vi "Launch DQMH Tools by menu.vi"(8 "error in":errorcluster, 11 "DQMH Tools":T1) -> (0 "error out":errorcluster)   [LabVIEW 2020]
doc: "Launch a DQMH scripting tool by typing one of the following strings in Quick Drop before pressing the Ctrl-Key shortcut for this plugin:\n\nCreate New DQMH Event - ae, new event, add event, create event, \"\" (empty string)\nRename DQMH Event - re, rename event\nRemove DQMH Event - rme, remove\nConvert DQMH Event - ce, convert\nAdd New DQMH Module - am, new mod, add mod, create mod\nRename DQMH Module - rm, rename module\nValidate DQMH Module - vm, validate\nCreate DQMH Module Template - ct, template\nCreate RT Tester - crt, rt\nNew DQMH Unit Test - cut, unit\n\nDefault Shortcut - [E]"
uses:
  controls/DQMH Tools Menu--enum.ctl
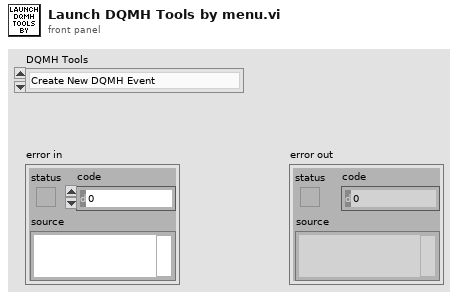
[diagram p1: front panel]
types:
  T1 = typedef "DQMH Tools Menu--enum.ctl" = enum16{"Create New DQMH Event", "Remove DQMH Event", "Convert DQMH Event", "Rename DQMH Event", "Add New DQMH Module", "Create RT Tester", "Rename DQMH Module", "Validate DQMH Module", "Create DQMH Module Template", "New DQMH  Unit Test"}
  T2 = enum32{"Invalid", "Standard", "Closed", "Hidden", "Minimized", "Maximized"}
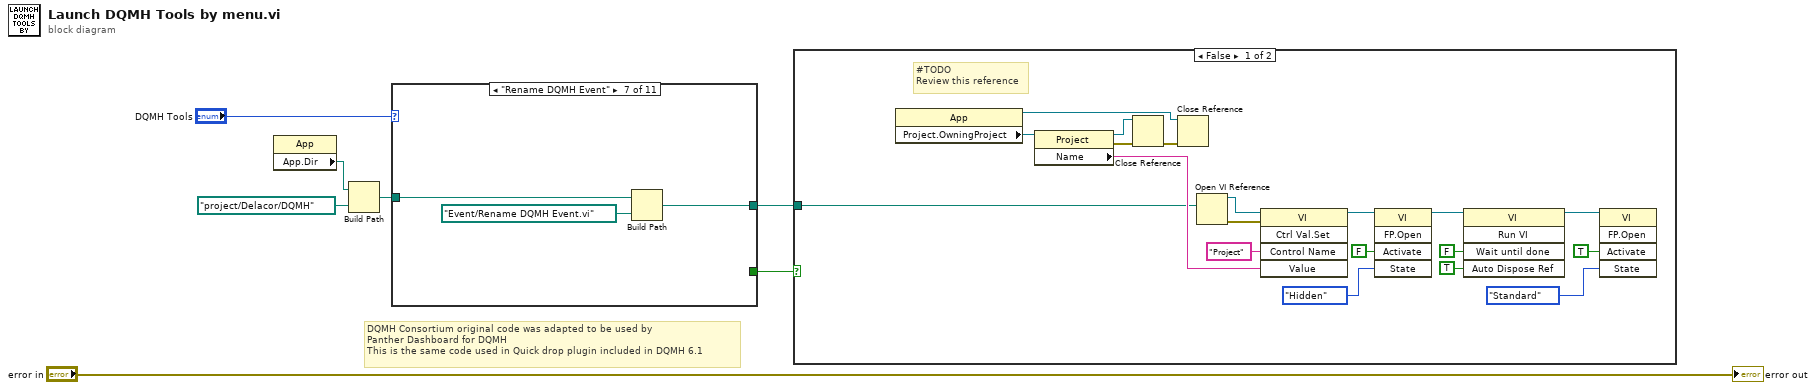
[diagram p0: block diagram]
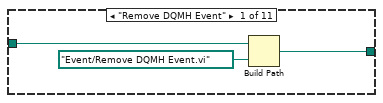
[diagram p3: hidden frame]
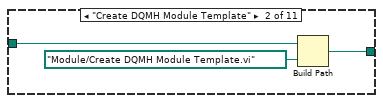
[diagram p4: hidden frame]
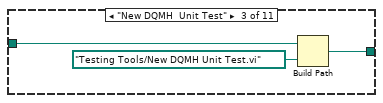
[diagram p5: hidden frame]
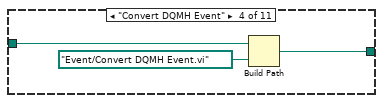
[diagram p6: hidden frame]
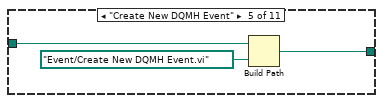
[diagram p7: hidden frame]
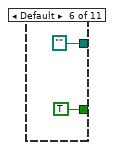
[diagram p8: hidden frame]
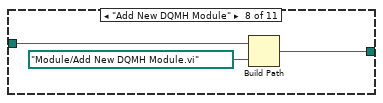
[diagram p9: hidden frame]
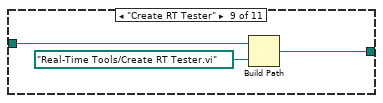
[diagram p10: hidden frame]
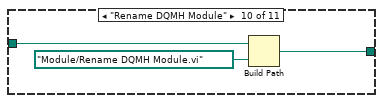
[diagram p11: hidden frame]
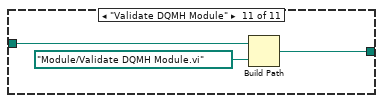
[diagram p12: hidden frame]
diagram:
  # "DQMH Consortium original code was adapted to be used by \nPanther Dashboard for DQMH\nThis is the same code used in Quick drop plugin included in DQMH 6.1"
  n1 = property class="App"() -> ("App.Dir"=w6:path)  [unwired: 2 in, 2 out]
  n2 = Build Path(base path=w6, name or relative path=path "project/Delacor/DQMH" ("Application:Directory Path")) -> (appended path=w4:path)
  n3 = case shown="\"Rename DQMH Event\"" "DQMH Tools" {
    tunnel: w4 -> [w10 w13 w16 w19 w22 _ w27 w30 w33 w36 w39]
    tunnel: [w9 w12 w15 w18 w21 path "" w26 w29 w32 w35 w38] -> w3
    tunnel: [_ _ _ _ _ TRUE _ _ _ _ _] -> w1
    frame "Remove DQMH Event" {
      n4 = Build Path(base path=w10, name or relative path=path "Event/Remove DQMH Event.vi") -> (appended path=w9:path)
    }
    frame "Create DQMH Module Template" {
      n5 = Build Path(base path=w13, name or relative path=path "Module/Create DQMH Module Template.vi") -> (appended path=w12:path)
    }
    frame "New DQMH  Unit Test" {
      n6 = Build Path(base path=w16, name or relative path=path "Testing Tools/New DQMH Unit Test.vi") -> (appended path=w15:path)
    }
    frame "Convert DQMH Event" {
      n7 = Build Path(base path=w19, name or relative path=path "Event/Convert DQMH Event.vi") -> (appended path=w18:path)
    }
    frame "Create New DQMH Event" {
      n8 = Build Path(base path=w22, name or relative path=path "Event/Create New DQMH Event.vi") -> (appended path=w21:path)
    }
    frame Default {
    }
    frame "Rename DQMH Event" {
      n9 = Build Path(base path=w27, name or relative path=path "Event/Rename DQMH Event.vi") -> (appended path=w26:path)
    }
    frame "Add New DQMH Module" {
      n10 = Build Path(base path=w30, name or relative path=path "Module/Add New DQMH Module.vi") -> (appended path=w29:path)
    }
    frame "Create RT Tester" {
      n11 = Build Path(base path=w33, name or relative path=path "Real-Time Tools/Create RT Tester.vi") -> (appended path=w32:path)
    }
    frame "Rename DQMH Module" {
      n12 = Build Path(base path=w36, name or relative path=path "Module/Rename DQMH Module.vi") -> (appended path=w35:path)
    }
    frame "Validate DQMH Module" {
      n13 = Build Path(base path=w39, name or relative path=path "Module/Validate DQMH Module.vi") -> (appended path=w38:path)
    }
  }
  n14 = case shown="False" w1 {
    tunnel: w3 -> [w47 _]
    frame False {
      # "#TODO\nReview this reference"
      n15 = property class="App"() -> (reference out=w48:refnum<vi>, "Project.OwningProject"=w51:refnum<vi>)  [unwired: 2 in, 1 out]
      n16 = property class="Project"(reference=w51) -> (reference out=w49:refnum<vi>, error out=w57:errorcluster, "Name"=w50:string)  [unwired: 1 in]
      n17 = Close Reference(reference=w49, error in (no error)=w57) -> (error out=w56:errorcluster)
      n18 = Close Reference(reference=w48, error in (no error)=w56) -> ()  [unwired: 1 out]
      n19 = Open VI Reference(vi path=w47) -> (vi reference=w55:refnum<vi>, error out=w58:errorcluster)  [unwired: 5 in]
      n20 = invoke class="VI" method="Ctrl Val.Set"(reference=w55, error in=w58, "Control Name"="Project", "Value"=w50) -> (reference out=w53:refnum<vi>)  [unwired: 1 in, 4 out]
      n21 = invoke class="VI" method="FP.Open"(reference=w53, "Activate"=FALSE ("Wait Until Done"), "State"=T2."Hidden") -> (reference out=w45:refnum<vi>)  [unwired: 2 in, 4 out]
      n22 = invoke class="VI" method="Run VI"(reference=w45, "Wait until done"=FALSE ("Wait Until Done"), "Auto Dispose Ref"=TRUE ("Auto Dispose Reference")) -> (reference out=w42:refnum<vi>)  [unwired: 2 in, 4 out]
      n23 = invoke class="VI" method="FP.Open"(reference=w42, "Activate"=TRUE ("Activate?"), "State"=T2."Standard") -> ()  [unwired: 2 in, 5 out]
    }
    frame True {
    }
  }
  "error out" <- "error in"
